vi "File_MakeTopLevel.vi"(1 "VI paths":path[](array[path]), 3 "TopLevel?":bool=TRUE, 5 "error in (no error)":errorcluster) -> (19 "error out":errorcluster)   [LabVIEW 2020]
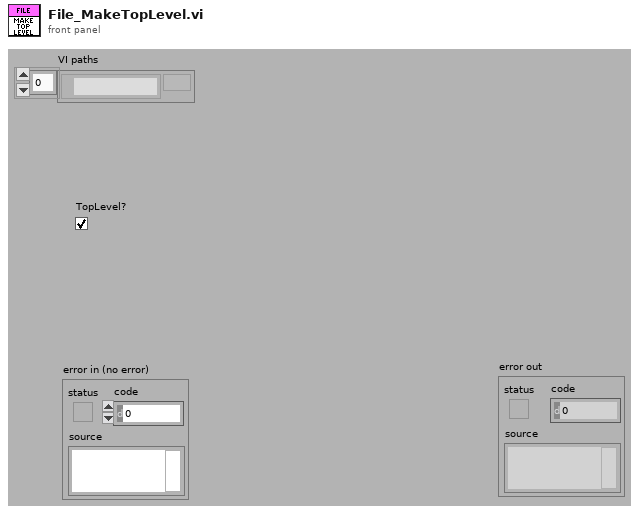
[diagram p1: front panel]
types:
  T1 = typedef "Librarian File Info Out.ctl" = cluster{"creation date":u32, "last mod date":u32, "type":string, "creator":string, "LV version":i32, "size":i32, "top level":bool}
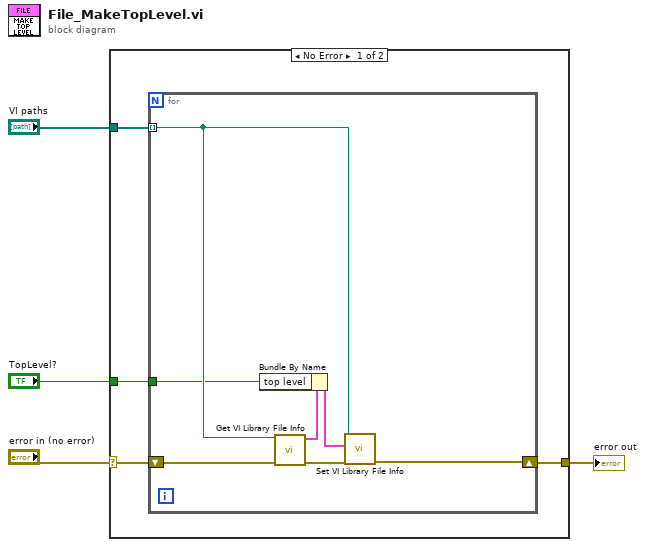
[diagram p0: block diagram]
diagram:
  n1 = case shown="No Error" "error in (no error)" {
    selector: "error in (no error)" -> [w8 w16]
    tunnel: "VI paths" -> [w7 _]
    tunnel: "TopLevel?" -> [w6 _]
    tunnel: [w5 w16] -> w1
    frame No Error {
      n2 = for {
        shift-right: [w15] -> w5
        shift-left: w8 -> [w13]
        tunnel: w7 -> [w10] mode=indexing
        tunnel: w6 -> [w9]
        n3 = call <vilib>:"Get VI Library File Info.vi"("error in (no error)"=w13, "path"=w10) -> ("error out"=w14:errorcluster, "file information"=w12:T1)  [unwired: 8 out]
        n4 = Bundle By Name(cluster=w12, "top level"=w9) -> (w11:T1)
        n5 = call <vilib>:"Set VI Library File Info.vi"("error in (no error)"=w14, "file information"=w11, "path"=w10) -> ("error out"=w15:errorcluster)  [unwired: 8 out]
      }
    }
    frame Error {
    }
  }
  "error out" <- w1
